vi "Lakeshore_370_write_only_readout.vi"(5 "File Reference":refnum<file>) -> ()   [LabVIEW 2019]
uses:
  Instrument_Setup.vi
  Global/Global Variables/global.vi
  Global/Global Variables/Data_Display_global.vi
panel:
  # "OFF"
  # "ON"
  # "OFF"
  # "ON"
  # "OFF"
  # "ON"
  # "OFF"
  # "ON"
  # "ON"
  # "OFF"
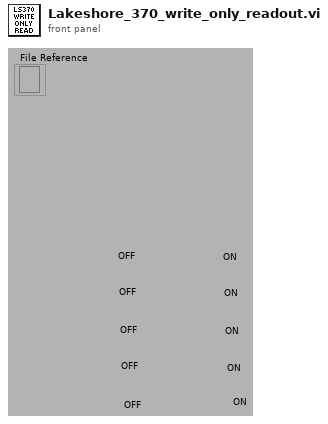
[diagram p1: front panel]
types:
  T1 = typedef "LS370_only_readout_cluster.ctl" = cluster{"LS370 T1":dbl, "LS370 T2":dbl, "LS370 T3":dbl, "LS370 T4":dbl, "LS370 T5":dbl, "LS370 R1":dbl, "LS370 R2":dbl, "LS370 R3":dbl, "LS370 R4":dbl, "LS370 R5":dbl, "LS370 T6":dbl, "LS370 T7":dbl, "LS370 T8":dbl, "LS370 T9":dbl, "LS370 R6":dbl, "LS370 R7":dbl, "LS370 R8":dbl, "LS370 R9":dbl, "LS370 TC-T":dbl, "LS370 TC-R":dbl, "Update Lakeshores":bool}
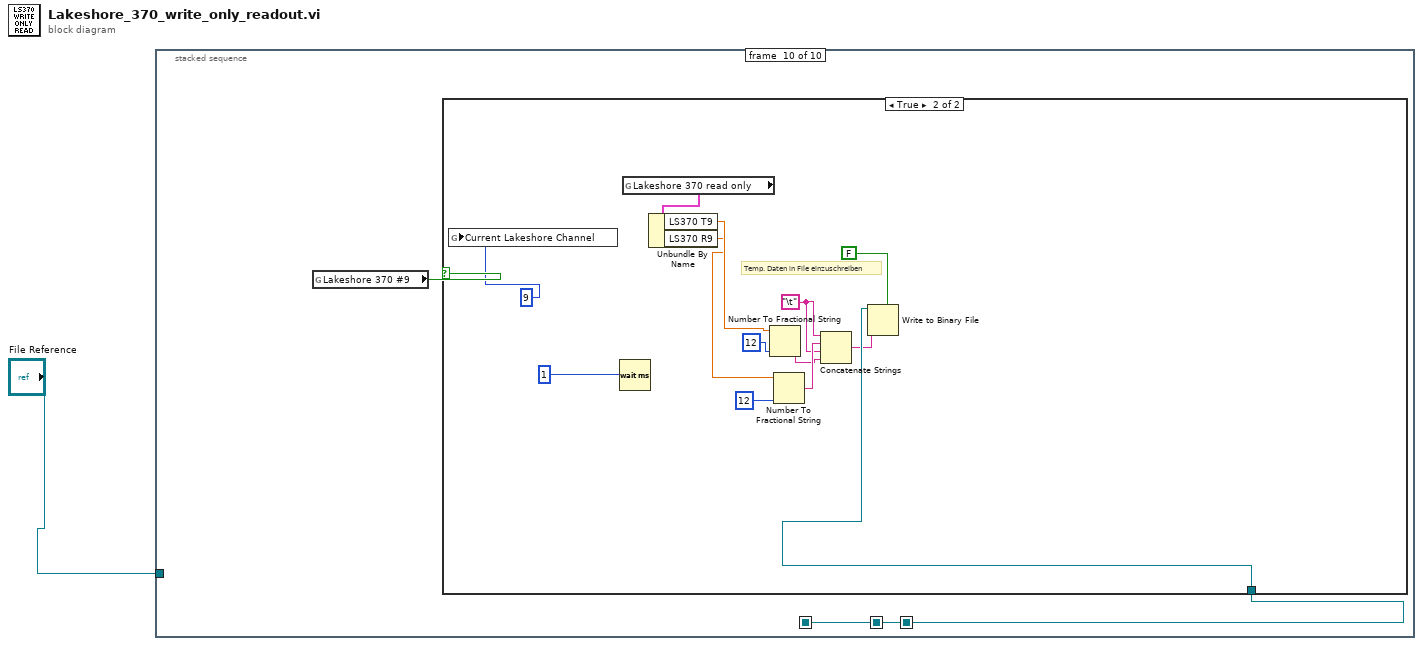
[diagram p0: block diagram]
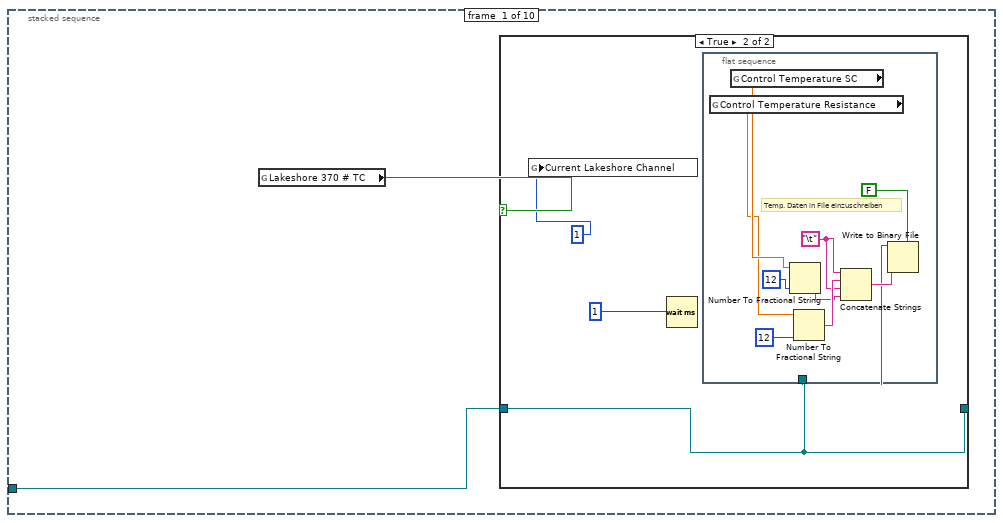
[diagram p2: hidden frame]
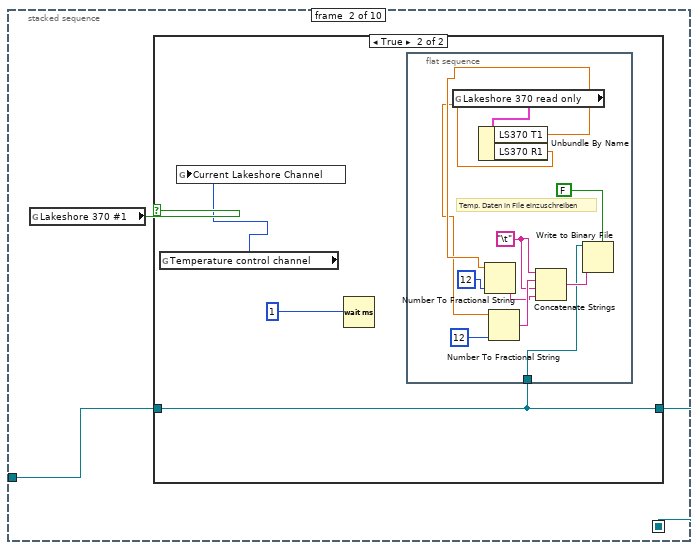
[diagram p4: hidden frame]
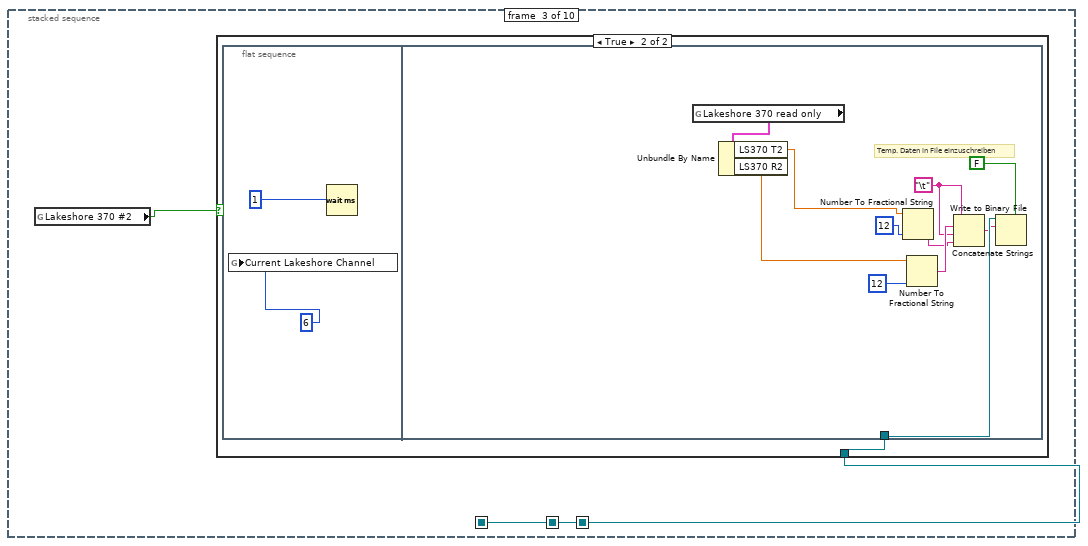
[diagram p6: hidden frame]
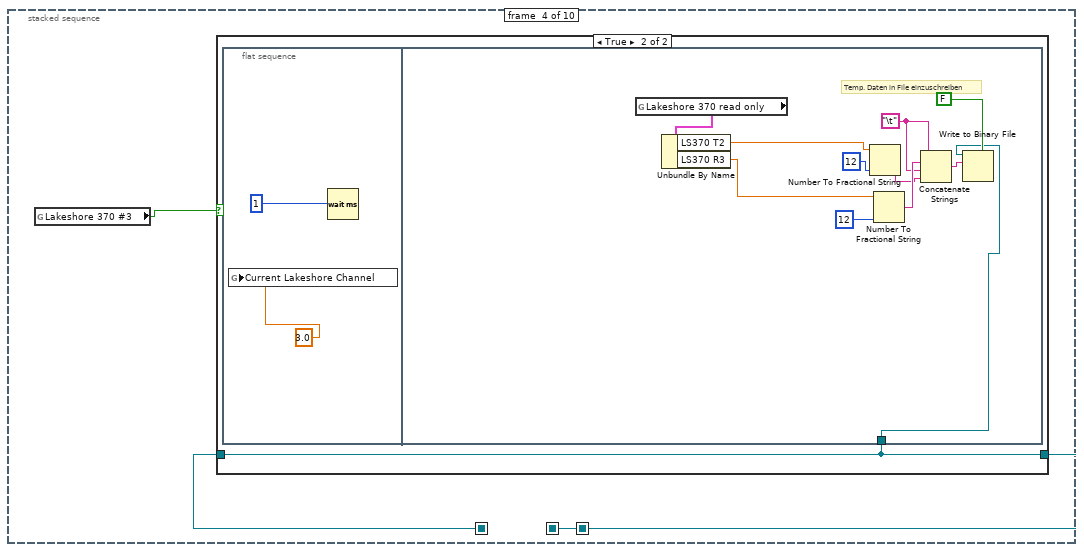
[diagram p8: hidden frame]
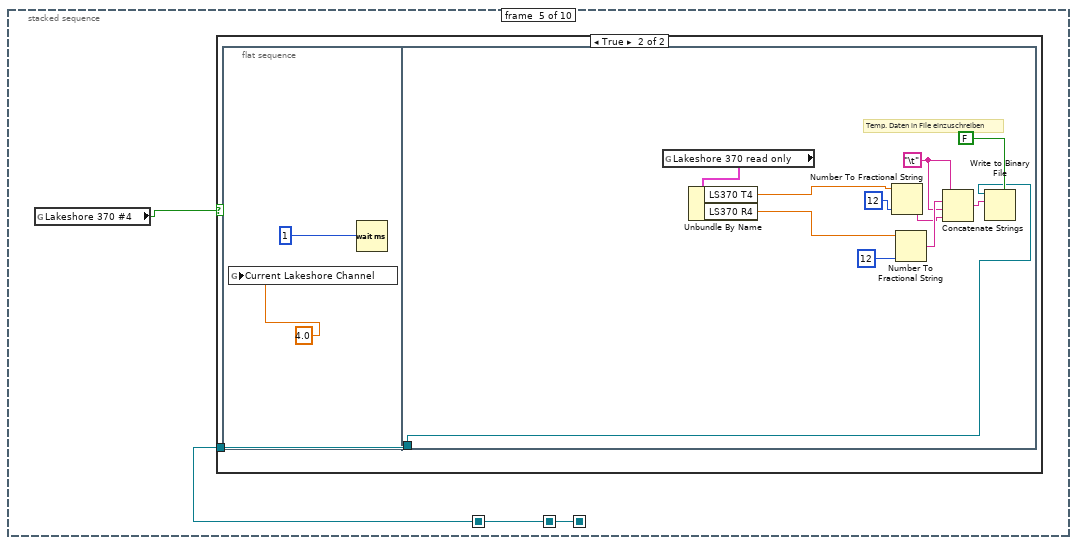
[diagram p10: hidden frame]
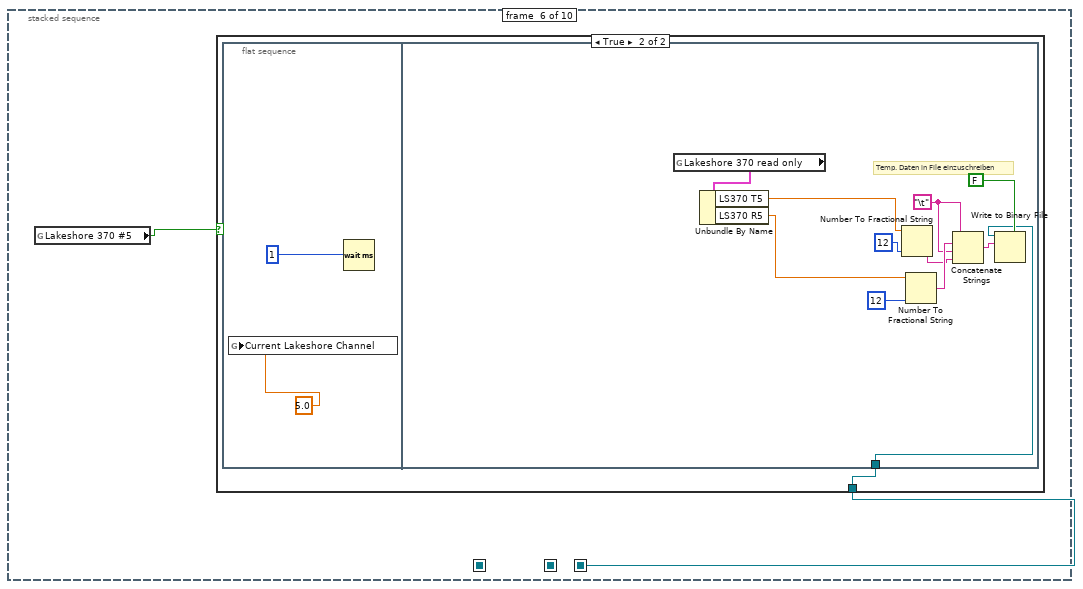
[diagram p12: hidden frame]
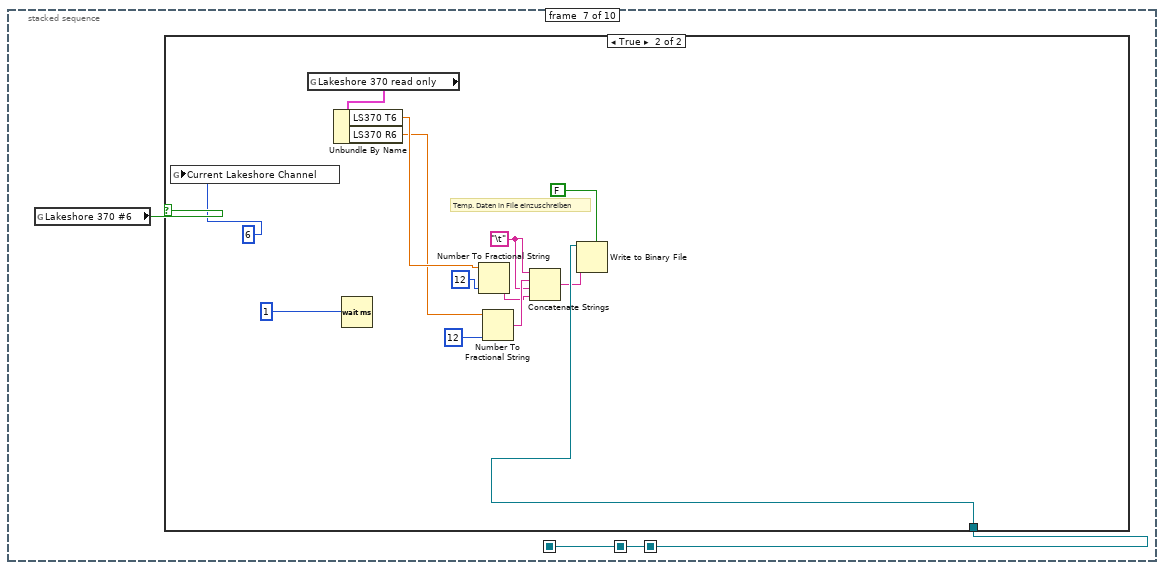
[diagram p14: hidden frame]
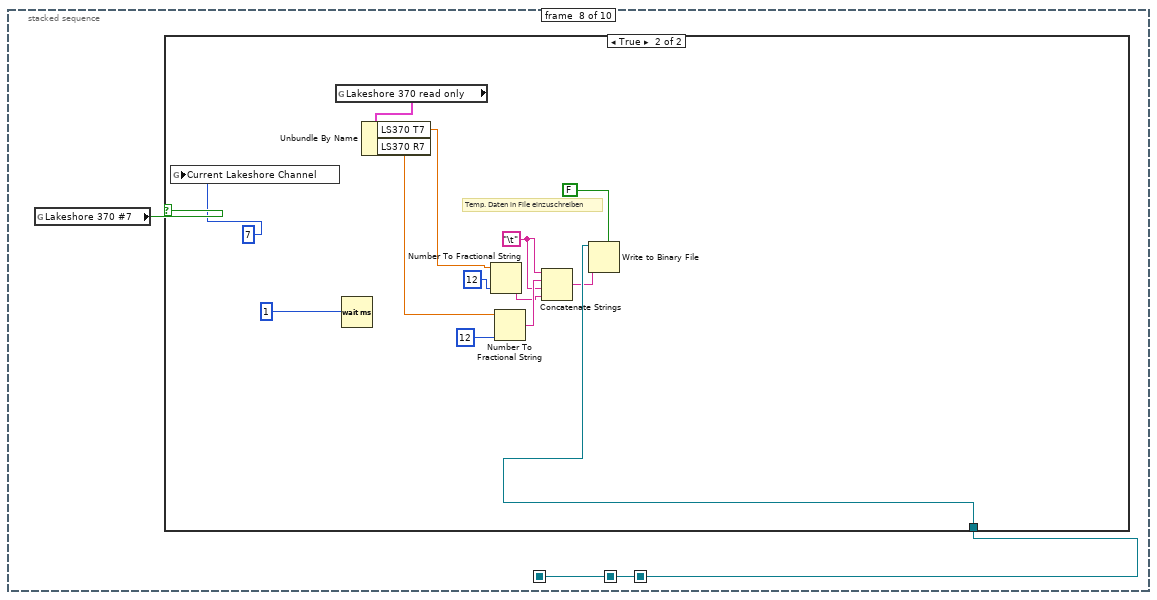
[diagram p16: hidden frame]
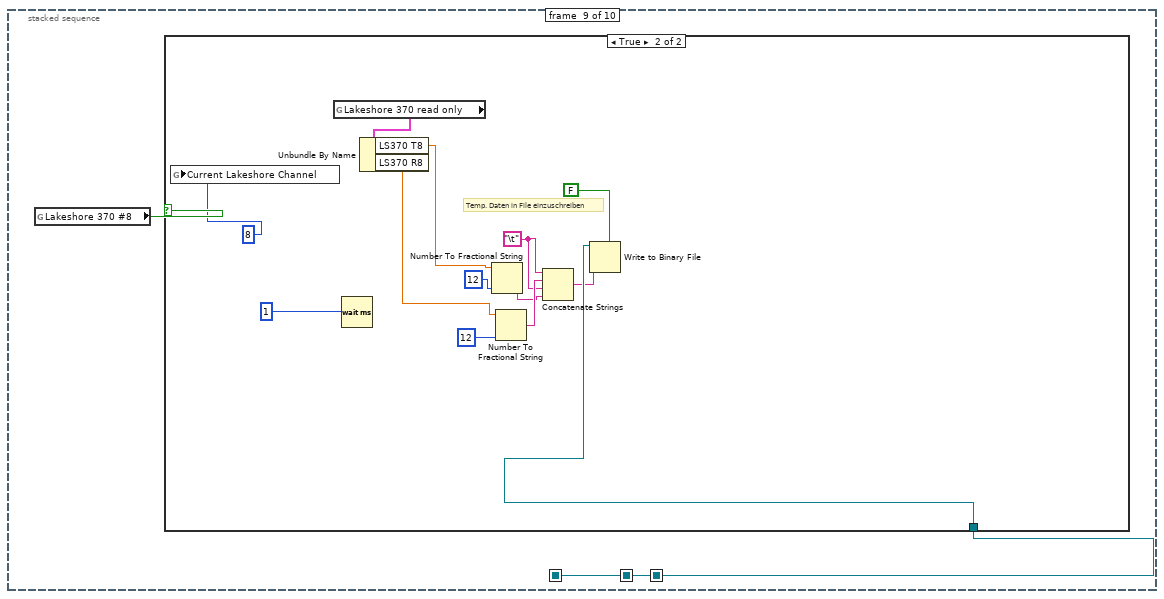
[diagram p18: hidden frame]
diagram:
  n1 = stacked-sequence {
    seq-local: [_ w19 _ _ _ _ _ _ _ _] -> [_ _ w36 w53 _ _ w102 w117 w132 w147]
    seq-local: [_ _ _ w52 _ _ _ _ _ _] -> [_ _ _ _ w70 _ _ _ _ _]
    seq-local: [_ _ _ _ w70 _ _ _ _ _] -> [_ _ _ _ _ w86 _ _ _ _]
    tunnel: "File Reference" -> [w2 w18 _ _ _ _ _ _ _ _]
    frame #0 {
      n2 = global read "Instrument_Setup.vi" "Lakeshore 370 # TC"() -> (w3:bool)
      n3 = case shown="True" w3 {
        tunnel: w2 -> [w4 w7]
        tunnel: [w4 w7] -> _
        frame False {
        }
        frame True {
          n4 = global write "global.vi" "Current Lakeshore Channel"(1) -> ()
          n5 = Wait (ms)(milliseconds to wait=1) -> ()  [unwired: 1 out]
          n6 = flat-sequence {
            tunnel: w7 -> [w13]
            frame #0 {
              w11 = "\t"
              # "Temp. Daten in File einzuschreiben"
              n7 = global read "Data_Display_global.vi" "Control Temperature Resistance"() -> (w8:dbl)
              n8 = global read "Data_Display_global.vi" "Control Temperature SC"() -> (w9:dbl)
              n9 = Number To Fractional String(number=w9, precision (6)=i16 12) -> (F-format string=w10:string)  [unwired: 2 in]
              n10 = Number To Fractional String(number=w8, precision (6)=i16 12) -> (F-format string=w16:string)  [unwired: 2 in]
              n11 = Concatenate Strings(w11, w16, w11, w10) -> (w17:string)
              n12 = Write to Binary File ("Write File")(file (use dialog)=w13, data=w17, 5:FALSE ("prepend array or string size? (T)")) -> ()  [unwired: 3 in, 3 out]
            }
          }
        }
      }
    }
    frame #1 {
      n13 = global read "Instrument_Setup.vi" "Lakeshore 370 #1"() -> (w20:bool)
      n14 = case shown="True" w20 {
        tunnel: w18 -> [w21 w23]
        tunnel: [w21 w23] -> w19
        frame False {
        }
        frame True {
          n15 = global read "Instrument_Setup.vi" "Temperature control channel"() -> (w22:i32)
          n16 = global write "global.vi" "Current Lakeshore Channel"(w22) -> ()
          n17 = Wait (ms)(milliseconds to wait=1) -> ()  [unwired: 1 out]
          n18 = flat-sequence {
            tunnel: w23 -> [w28]
            frame #0 {
              w30 = "\t"
              # "Temp. Daten in File einzuschreiben"
              n19 = global read "Data_Display_global.vi" "Lakeshore 370 read only"() -> (w27:T1)
              n20 = Unbundle By Name(w27) -> ("LS370 T1"=w26:dbl, "LS370 R1"=w25:dbl)
              n21 = Number To Fractional String(number=w26, precision (6)=i16 12) -> (F-format string=w29:string)  [unwired: 2 in]
              n22 = Number To Fractional String(number=w25, precision (6)=i16 12) -> (F-format string=w34:string)  [unwired: 2 in]
              n23 = Concatenate Strings(w30, w34, w30, w29) -> (w35:string)
              n24 = Write to Binary File ("Write File")(file (use dialog)=w28, data=w35, 5:FALSE ("prepend array or string size? (T)")) -> ()  [unwired: 3 in, 3 out]
            }
          }
        }
      }
    }
    frame #2 {
      n25 = global read "Instrument_Setup.vi" "Lakeshore 370 #2"() -> (w37:bool)
      n26 = case shown="True" w37 {
        tunnel: w36 -> [_ w38]
        frame False {
        }
        frame True {
          n27 = flat-sequence {
            tunnel: w38 -> [w50]
            frame #0 {
              n28 = global write "global.vi" "Current Lakeshore Channel"(6) -> ()
              n29 = Wait (ms)(milliseconds to wait=1) -> ()  [unwired: 1 out]
            }
            frame #1 {
              w46 = "\t"
              # "Temp. Daten in File einzuschreiben"
              n30 = global read "Data_Display_global.vi" "Lakeshore 370 read only"() -> (w43:T1)
              n31 = Unbundle By Name(w43) -> ("LS370 T2"=w42:dbl, "LS370 R2"=w41:dbl)
              n32 = Number To Fractional String(number=w42, precision (6)=i16 12) -> (F-format string=w45:string)  [unwired: 2 in]
              n33 = Number To Fractional String(number=w41, precision (6)=i16 12) -> (F-format string=w49:string)  [unwired: 2 in]
              n34 = Concatenate Strings(w46, w49, w46, w45) -> (w44:string)
              n35 = Write to Binary File ("Write File")(file (use dialog)=w50, data=w44, 5:FALSE ("prepend array or string size? (T)")) -> ()  [unwired: 3 in, 3 out]
            }
          }
        }
      }
    }
    frame #3 {
      n36 = global read "Instrument_Setup.vi" "Lakeshore 370 #3"() -> (w54:bool)
      n37 = case shown="True" w54 {
        tunnel: w53 -> [w55 w56]
        tunnel: [w55 w56] -> w52
        frame False {
        }
        frame True {
          n38 = flat-sequence {
            tunnel: w56 -> [w62]
            frame #0 {
              n39 = global write "global.vi" "Current Lakeshore Channel"(3.0) -> ()
              n40 = Wait (ms)(milliseconds to wait=1) -> ()  [unwired: 1 out]
            }
            frame #1 {
              w65 = "\t"
              # "Temp. Daten in File einzuschreiben"
              n41 = global read "Data_Display_global.vi" "Lakeshore 370 read only"() -> (w61:T1)
              n42 = Unbundle By Name(w61) -> ("LS370 T2"=w60:dbl, "LS370 R3"=w59:dbl)
              n43 = Number To Fractional String(number=w60, precision (6)=i16 12) -> (F-format string=w64:string)  [unwired: 2 in]
              n44 = Number To Fractional String(number=w59, precision (6)=i16 12) -> (F-format string=w68:string)  [unwired: 2 in]
              n45 = Concatenate Strings(w65, w68, w65, w64) -> (w63:string)
              n46 = Write to Binary File ("Write File")(file (use dialog)=w62, data=w63, 5:FALSE ("prepend array or string size? (T)")) -> ()  [unwired: 3 in, 3 out]
            }
          }
        }
      }
    }
    frame #4 {
      n47 = global read "Instrument_Setup.vi" "Lakeshore 370 #4"() -> (w71:bool)
      n48 = case shown="True" w71 {
        tunnel: w70 -> [_ w72]
        frame False {
        }
        frame True {
          n49 = flat-sequence {
            tunnel: w72 -> [w78]
            frame #0 {
              n50 = global write "global.vi" "Current Lakeshore Channel"(4.0) -> ()
              n51 = Wait (ms)(milliseconds to wait=1) -> ()  [unwired: 1 out]
            }
            frame #1 {
              w81 = "\t"
              # "Temp. Daten in File einzuschreiben"
              n52 = global read "Data_Display_global.vi" "Lakeshore 370 read only"() -> (w77:T1)
              n53 = Unbundle By Name(w77) -> ("LS370 T4"=w76:dbl, "LS370 R4"=w75:dbl)
              n54 = Number To Fractional String(number=w76, precision (6)=i16 12) -> (F-format string=w80:string)  [unwired: 2 in]
              n55 = Number To Fractional String(number=w75, precision (6)=i16 12) -> (F-format string=w84:string)  [unwired: 2 in]
              n56 = Concatenate Strings(w81, w84, w81, w80) -> (w79:string)
              n57 = Write to Binary File ("Write File")(file (use dialog)=w78, data=w79, 5:FALSE ("prepend array or string size? (T)")) -> ()  [unwired: 3 in, 3 out]
            }
          }
        }
      }
    }
    frame #5 {
      n58 = global read "Instrument_Setup.vi" "Lakeshore 370 #5"() -> (w87:bool)
      n59 = case shown="True" w87 {
        tunnel: w86 -> [_ w88]
        frame False {
        }
        frame True {
          n60 = flat-sequence {
            tunnel: w88 -> [w94]
            frame #0 {
              n61 = global write "global.vi" "Current Lakeshore Channel"(5.0) -> ()
              n62 = Wait (ms)(milliseconds to wait=1) -> ()  [unwired: 1 out]
            }
            frame #1 {
              w97 = "\t"
              # "Temp. Daten in File einzuschreiben"
              n63 = global read "Data_Display_global.vi" "Lakeshore 370 read only"() -> (w93:T1)
              n64 = Unbundle By Name(w93) -> ("LS370 T5"=w92:dbl, "LS370 R5"=w91:dbl)
              n65 = Number To Fractional String(number=w92, precision (6)=i16 12) -> (F-format string=w96:string)  [unwired: 2 in]
              n66 = Number To Fractional String(number=w91, precision (6)=i16 12) -> (F-format string=w100:string)  [unwired: 2 in]
              n67 = Concatenate Strings(w97, w100, w97, w96) -> (w95:string)
              n68 = Write to Binary File ("Write File")(file (use dialog)=w94, data=w95, 5:FALSE ("prepend array or string size? (T)")) -> ()  [unwired: 3 in, 3 out]
            }
          }
        }
      }
    }
    frame #6 {
      n69 = global read "Instrument_Setup.vi" "Lakeshore 370 #6"() -> (w103:bool)
      n70 = case shown="True" w103 {
        tunnel: w102 -> [_ w114]
        frame False {
        }
        frame True {
          w108 = "\t"
          # "Temp. Daten in File einzuschreiben"
          n71 = global write "global.vi" "Current Lakeshore Channel"(6) -> ()
          n72 = global read "Data_Display_global.vi" "Lakeshore 370 read only"() -> (w106:T1)
          n73 = Unbundle By Name(w106) -> ("LS370 T6"=w105:dbl, "LS370 R6"=w104:dbl)
          n74 = Wait (ms)(milliseconds to wait=1) -> ()  [unwired: 1 out]
          n75 = Number To Fractional String(number=w105, precision (6)=i16 12) -> (F-format string=w107:string)  [unwired: 2 in]
          n76 = Number To Fractional String(number=w104, precision (6)=i16 12) -> (F-format string=w112:string)  [unwired: 2 in]
          n77 = Concatenate Strings(w108, w112, w108, w107) -> (w113:string)
          n78 = Write to Binary File ("Write File")(file (use dialog)=w114, data=w113, 5:FALSE ("prepend array or string size? (T)")) -> ()  [unwired: 3 in, 3 out]
        }
      }
    }
    frame #7 {
      n79 = global read "Instrument_Setup.vi" "Lakeshore 370 #7"() -> (w118:bool)
      n80 = case shown="True" w118 {
        tunnel: w117 -> [_ w129]
        frame False {
        }
        frame True {
          w123 = "\t"
          # "Temp. Daten in File einzuschreiben"
          n81 = global write "global.vi" "Current Lakeshore Channel"(7) -> ()
          n82 = global read "Data_Display_global.vi" "Lakeshore 370 read only"() -> (w121:T1)
          n83 = Wait (ms)(milliseconds to wait=1) -> ()  [unwired: 1 out]
          n84 = Unbundle By Name(w121) -> ("LS370 T7"=w120:dbl, "LS370 R7"=w119:dbl)
          n85 = Number To Fractional String(number=w120, precision (6)=i16 12) -> (F-format string=w122:string)  [unwired: 2 in]
          n86 = Number To Fractional String(number=w119, precision (6)=i16 12) -> (F-format string=w127:string)  [unwired: 2 in]
          n87 = Concatenate Strings(w123, w127, w123, w122) -> (w128:string)
          n88 = Write to Binary File ("Write File")(file (use dialog)=w129, data=w128, 5:FALSE ("prepend array or string size? (T)")) -> ()  [unwired: 3 in, 3 out]
        }
      }
    }
    frame #8 {
      n89 = global read "Instrument_Setup.vi" "Lakeshore 370 #8"() -> (w133:bool)
      n90 = case shown="True" w133 {
        tunnel: w132 -> [_ w144]
        frame False {
        }
        frame True {
          w138 = "\t"
          # "Temp. Daten in File einzuschreiben"
          n91 = global write "global.vi" "Current Lakeshore Channel"(8) -> ()
          n92 = global read "Data_Display_global.vi" "Lakeshore 370 read only"() -> (w136:T1)
          n93 = Wait (ms)(milliseconds to wait=1) -> ()  [unwired: 1 out]
          n94 = Unbundle By Name(w136) -> ("LS370 T8"=w135:dbl, "LS370 R8"=w134:dbl)
          n95 = Number To Fractional String(number=w135, precision (6)=i16 12) -> (F-format string=w137:string)  [unwired: 2 in]
          n96 = Number To Fractional String(number=w134, precision (6)=i16 12) -> (F-format string=w142:string)  [unwired: 2 in]
          n97 = Concatenate Strings(w138, w142, w138, w137) -> (w143:string)
          n98 = Write to Binary File ("Write File")(file (use dialog)=w144, data=w143, 5:FALSE ("prepend array or string size? (T)")) -> ()  [unwired: 3 in, 3 out]
        }
      }
    }
    frame #9 {
      n99 = global read "Instrument_Setup.vi" "Lakeshore 370 #9"() -> (w148:bool)
      n100 = case shown="True" w148 {
        tunnel: w147 -> [_ w159]
        frame False {
        }
        frame True {
          w153 = "\t"
          # "Temp. Daten in File einzuschreiben"
          n101 = global write "global.vi" "Current Lakeshore Channel"(9) -> ()
          n102 = Wait (ms)(milliseconds to wait=1) -> ()  [unwired: 1 out]
          n103 = global read "Data_Display_global.vi" "Lakeshore 370 read only"() -> (w151:T1)
          n104 = Unbundle By Name(w151) -> ("LS370 T9"=w150:dbl, "LS370 R9"=w149:dbl)
          n105 = Number To Fractional String(number=w150, precision (6)=i16 12) -> (F-format string=w152:string)  [unwired: 2 in]
          n106 = Number To Fractional String(number=w149, precision (6)=i16 12) -> (F-format string=w157:string)  [unwired: 2 in]
          n107 = Concatenate Strings(w153, w157, w153, w152) -> (w158:string)
          n108 = Write to Binary File ("Write File")(file (use dialog)=w159, data=w158, 5:FALSE ("prepend array or string size? (T)")) -> ()  [unwired: 3 in, 3 out]
        }
      }
    }
  }
